vi "Update Number of Steps Tree Tag.vi"(10 "New Number of Steps":i32, 11 "TreeControl in":refnum<vi>) -> (3 "TreeControl out":refnum<vi>)   [LabVIEW 2020, in "Output Sequencer.lvlib" / "Settings UI.lvclass"]
uses:
  Settings UI.lvclass
  Types/Tree Index Enum.ctl
  Globals/Global Tree Data.vi
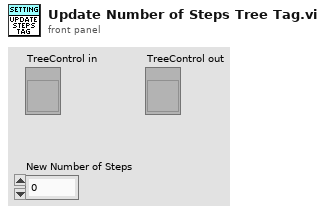
[diagram p1: front panel]
types:
  T1 = typedef "Output Sequencer.lvlib/Settings UI.lvclass/Tree Index Enum.ctl" = enum16{"General Settings", "Num Steps", "Num Analog", "Num Digital", "Show Confirmation", "Interp Priority", "Adv Timing", "Enable Conditions", "Seq Execution", "Reset Test Start", "Only When Test", "Delay After Test", "Start condition", "Re-triggering", "Stop condition", "Stop After Cycles", "Stop Values", "Default Values", "Default Analog", "Default Digital", "Steps", "Step #", "Description", "Precondition", "Duration", "Mode", "Delay Between Vals", "Analog Values", "Digital Values", "Postcondition", "On True", "On False"}
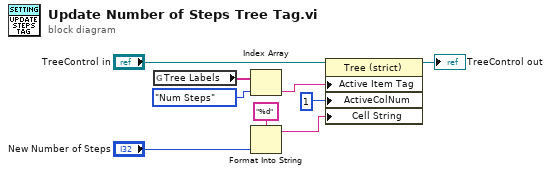
[diagram p0: block diagram]
diagram:
  n1 = global read "Global Tree Data.vi" "Tree Labels"() -> (w2:string[])
  n2 = Index Array(array=w2, index=Tree_Index_Enum."Num Steps" ("Tree Index Enum")) -> (element=w6:string)
  n3 = Format Into String(format string="%d", "New Number of Steps") -> (resulting string=w5:string)  [unwired: 2 in, 1 out]
  n4 = property class="Tree (strict)"(reference="TreeControl in", "Active Item Tag"=w6, "ActiveColNum"=1 ("Active Cell:Active Column Number"), "Cell String"=w5) -> (reference out=→"TreeControl out":refnum<vi>)  [unwired: 1 in, 1 out]
